vi "KeyenceCVX.Main-Scan.vi"(8 "error in":errorcluster, 10 "restart (T)":bool=TRUE) -> (0 "error out":errorcluster)   [LabVIEW 2016]
uses:
  KeyenceCVX.Action.ctl
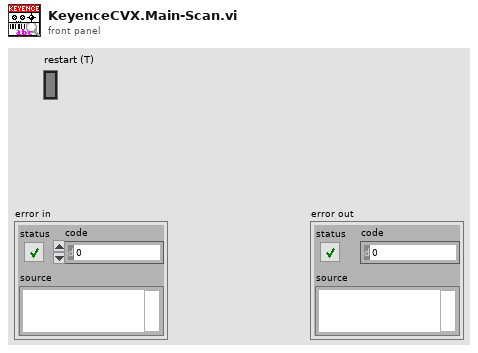
[diagram p1: front panel]
types:
  T1 = typedef "KeyenceCVX.Action.ctl" = enum32{"idle", "constructor", "destructor", "-- Keyence CVX --", "Init", "Scan", "ChangeProgram"}
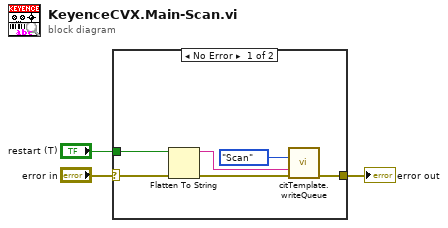
[diagram p0: block diagram]
diagram:
  n1 = case shown="No Error" "error in" {
    selector: "error in" -> [w9 w10]
    tunnel: [w8 w10] -> w2
    tunnel: "restart (T)" -> [w6 _]
    frame No Error {
      n2 = Flatten To String(anything=w6, error in (no error)=w9) -> (data string=w5:string, error out=w7:errorcluster)  [unwired: 2 in, 1 out]
      n3 = call "citTemplate.writeQueue.vi"("event in (if not connected:all statemachine with data event)"=KeyenceCVX.Action."Scan" ("Action"), "data in"=w5, "error in (no error)"=w7) -> ("error out"=w8:errorcluster)  [unwired: 12 in]
    }
    frame Error {
    }
  }
  "error out" <- w2
